vi "Unit Test.vi"() -> ()   [LabVIEW 2019, in "Allmotion.lvlib"]
uses:
  Allmotion.lvlib
  User Event/Controls/UE Abort Action.ctl
panel:
  in  "Open":bool
  out "Event":string
  in  "Current Position":i32[](array[numeric])
  in  "EMC Stop":bool
  in  "Joystick":bool
  in  "Reset":bool
  in  "Position":bool
  in  "Move":bool
  in  "Home":bool
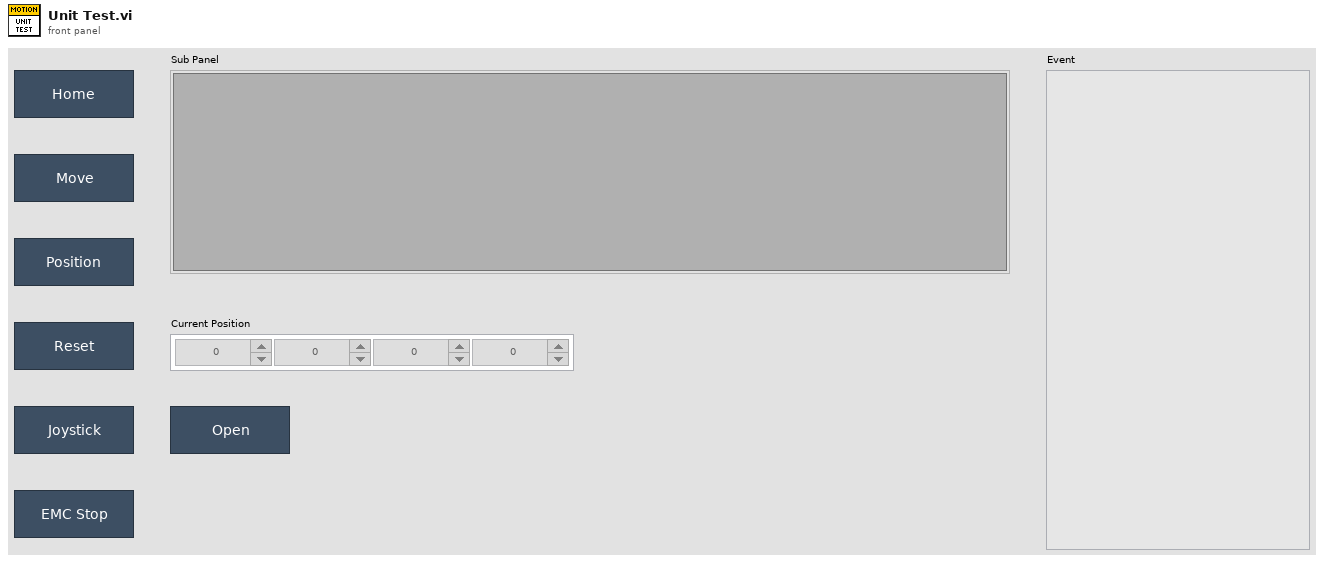
[diagram p1: front panel]
types:
  T1 = cluster{"Position":i32[], "Event":string, "Control Ref":refnum<vi>}
  T2 = typedef "UE Abort Action.ctl" = enum16{"Create", "Get", "Destroy"}
  T3 = typedef "Allmotion.lvlib/SEQ Data.ctl" = cluster{"Position":i32[], "Arrived?":bool, "VISA name":refnum<visa-resource-name>, "Initialize Done?":bool, "State":string, "VI Refnum":refnum<vi>, "Dichroic Position":string[]}
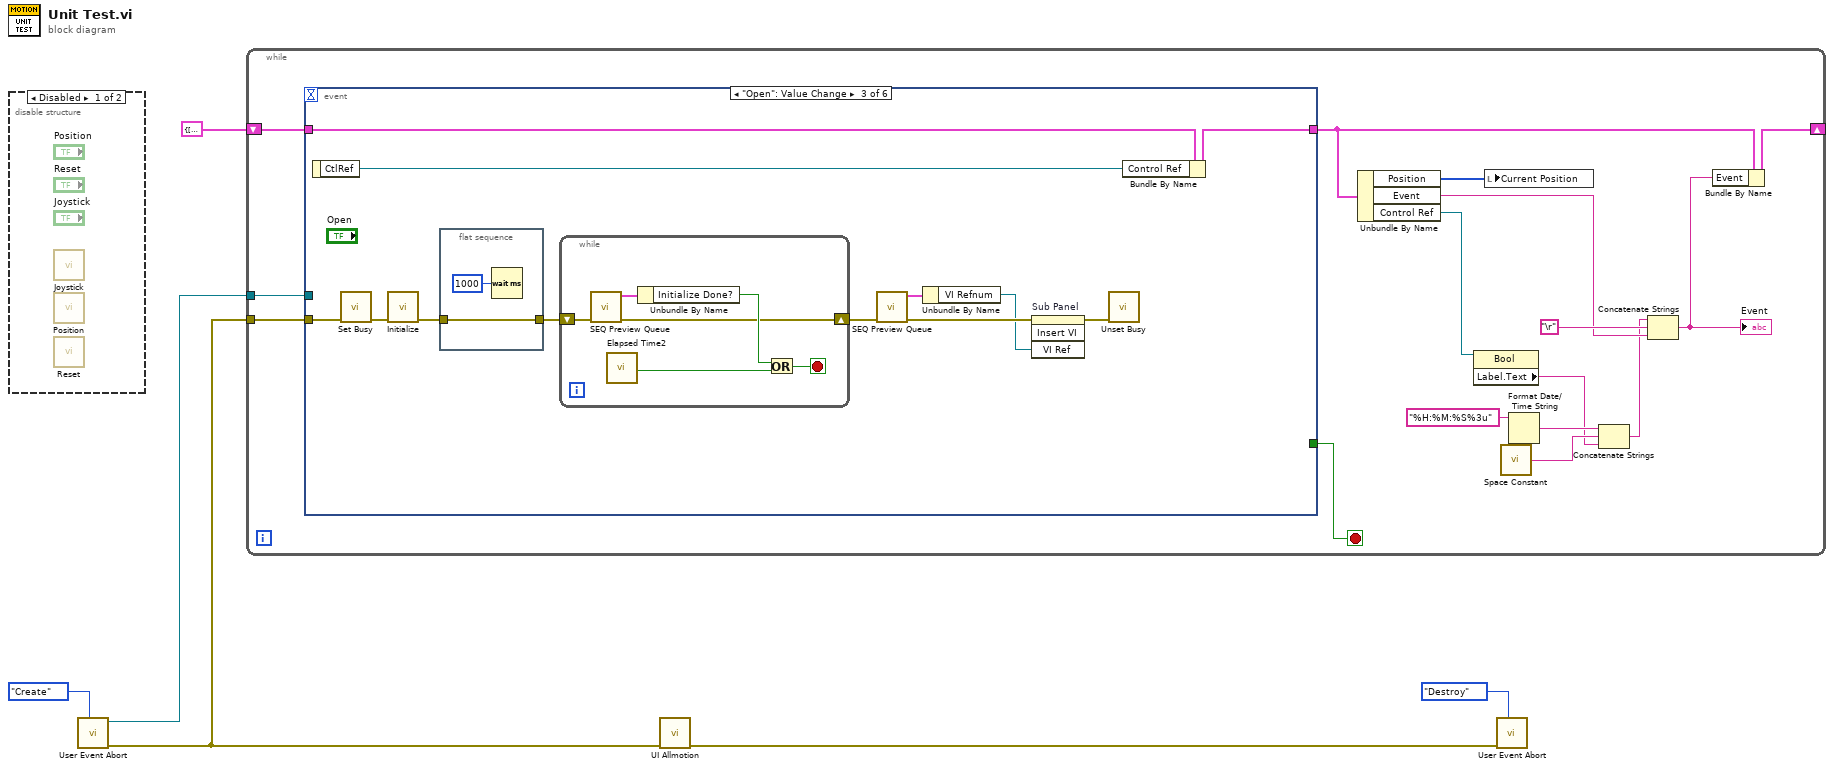
[diagram p0: block diagram]
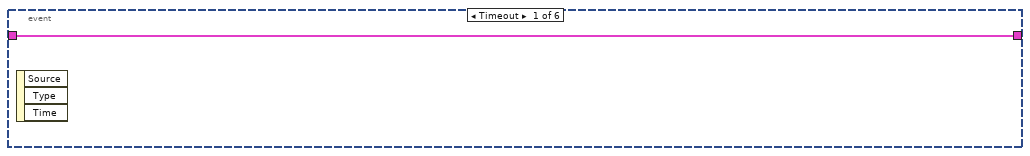
[diagram p3: hidden frame]
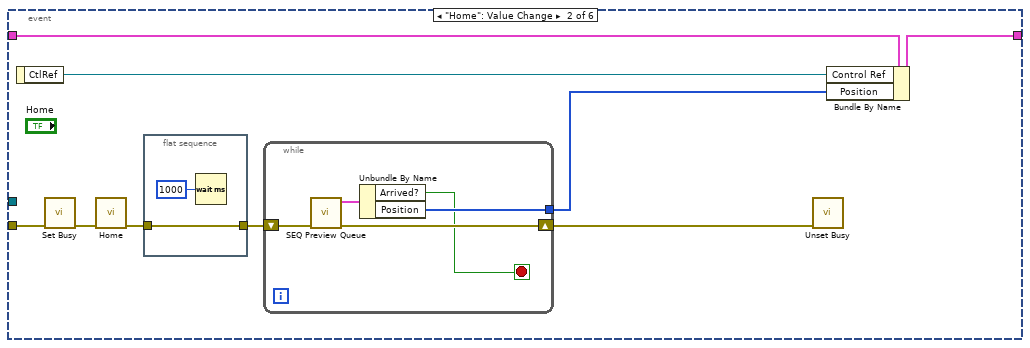
[diagram p4: hidden frame]
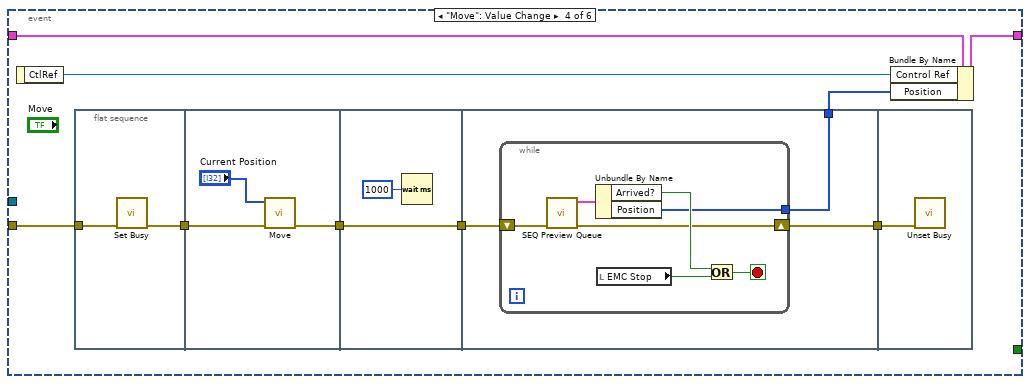
[diagram p5: hidden frame]
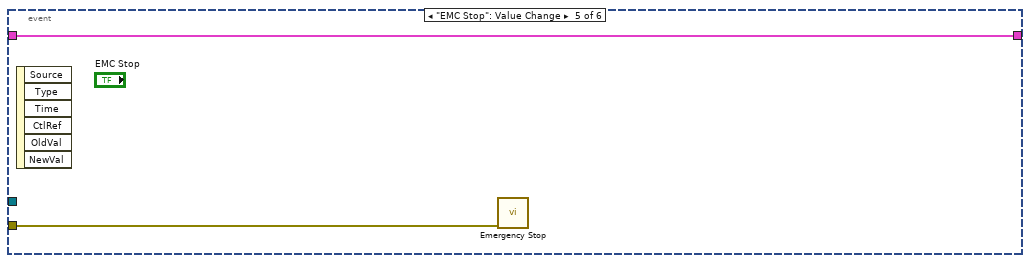
[diagram p6: hidden frame]
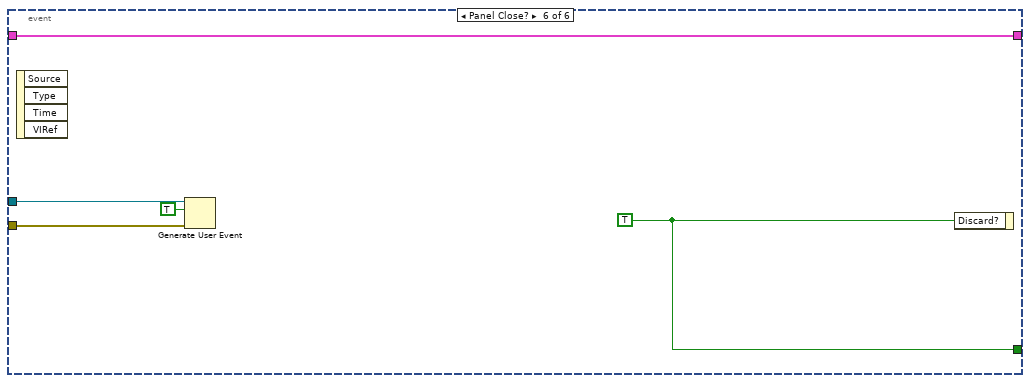
[diagram p7: hidden frame]
diagram:
  n1 = disable-structure shown="Disabled" {
    frame Disabled {
      n2 = call "Joystick.vi"() -> ()  [unwired: 11 in, 1 out]
      n3 = call "Position.vi"() -> ()  [unwired: 11 in, 1 out]
      n4 = call "Reset.vi"() -> ()  [unwired: 11 in, 1 out]
    }
    frame Enabled {
    }
  }
  n5 = call "User Event Abort.vi"("Action"=UE_Abort_Action."Create") -> ("Error Out"=w4:errorcluster, "User Event Out"=w5:refnum<user-event>)  [unwired: 9 in]
  n6 = while {
    tunnel: w5 -> [w21]
    tunnel: w4 -> [w20]
    shift-right: [w15] -> _
    shift-left: T1 {"Position"=[], "Event"="", "Control Ref"=refnum} -> [w19]
    stop <- w22 stop-if-true
    n7 = event shown="[2] \"Open\": Value Change" {
      selector: _ -> [_ _ _ _ _ _]
      dyn-events: _ -> [_ _ _ _ _ _]
      timeout: _ -> [_ _ _ _ _ _]
      tunnel: [_ _ _ _ _ w93] -> w22
      tunnel: w21 -> [_ _ _ _ _ w92]
      tunnel: w20 -> [_ w32 w51 w68 w87 w90]
      tunnel: w19 -> [w23 w30 w50 w64 w88 w89]
      tunnel: [w23 w29 w49 w63 w88 w89] -> w18
      event Timeout {
        n8 = event-data() -> ()  [unwired: 1 in, 3 out]
      }
      event "Home": Value Change {
        n9 = event-data() -> ("CtlRef"=w28:refnum<vi>)  [unwired: 1 in]
        n10 = call <vilib>:"Set Busy.vi"("error in (no error)"=w32) -> ("error out"=w31:errorcluster)  [unwired: 9 in, 1 out]
        n11 = call "Home.vi"("Error In"=w31) -> ("Error Out"=w26:errorcluster)  [unwired: 10 in]
        n12 = flat-sequence {
          tunnel: w26 -> [w33]
          tunnel: [w33] -> w25
          frame #0 {
            n13 = Wait (ms)(milliseconds to wait=u32 1000) -> ()  [unwired: 1 out]
          }
        }
        n14 = while {
          tunnel: [w37] -> w27
          shift-right: [w36] -> w24
          shift-left: w25 -> [w39]
          stop <- w35 stop-if-true
          n15 = call "SEQ Preview Queue.vi"("error in"=w39) -> ("error out"=w36:errorcluster, "SEQ Data"=w38:T3)  [unwired: 9 in]
          n16 = Unbundle By Name(w38) -> ("Arrived?"=w35:bool, "Position"=w37:i32[])
        }
        n17 = call <vilib>:"Unset Busy.vi"("error in (no error)"=w24) -> ()  [unwired: 10 in, 1 out]
        n18 = Bundle By Name(cluster=w30, "Control Ref"=w28, "Position"=w27) -> (w29:T1)
      }
      event "Open": Value Change {
        n19 = event-data() -> ("CtlRef"=w48:refnum<vi>)  [unwired: 1 in]
        n20 = call <vilib>:"Set Busy.vi"("error in (no error)"=w51) -> ("error out"=w42:errorcluster)  [unwired: 9 in, 1 out]
        n21 = call "Initialize.vi"("Error In"=w42) -> ("Error Out"=w41:errorcluster)  [unwired: 10 in]
        n22 = flat-sequence {
          tunnel: w41 -> [w52]
          tunnel: [w52] -> w40
          frame #0 {
            n23 = Wait (ms)(milliseconds to wait=u32 1000) -> ()  [unwired: 1 out]
          }
        }
        n24 = while {
          shift-right: [w55] -> w47
          shift-left: w40 -> [w59]
          stop <- w57 stop-if-true
          n25 = call "SEQ Preview Queue.vi"("error in"=w59) -> ("error out"=w55:errorcluster, "SEQ Data"=w58:T3)  [unwired: 9 in]
          n26 = call "Elapsed Time2"() -> ("Time has Elapsed"=w54:bool)  [unwired: 12 in, 7 out]
          n27 = Unbundle By Name(w58) -> ("Initialize Done?"=w56:bool)
          n28 = Or(x=w56, y=w54) -> (x .or. y?=w57:bool)
        }
        n29 = call "SEQ Preview Queue.vi"("error in"=w47) -> ("error out"=w45:errorcluster, "SEQ Data"=w46:T3)  [unwired: 9 in]
        n30 = Unbundle By Name(w46) -> ("VI Refnum"=w43:refnum<vi>)
        n31 = invoke on="Sub Panel" class="SubPnl" method="Insert VI"(error in=w45, "VI Ref"=w43) -> (error out=w44:errorcluster)  [unwired: 2 in, 3 out]
        n32 = call <vilib>:"Unset Busy.vi"("error in (no error)"=w44) -> ()  [unwired: 10 in, 1 out]
        n33 = Bundle By Name(cluster=w50, "Control Ref"=w48) -> (w49:T1)
      }
      event "Move": Value Change {
        n34 = event-data() -> ("CtlRef"=w62:refnum<vi>)  [unwired: 1 in]
        n35 = flat-sequence {
          tunnel: w68 -> [w70]
          tunnel: [w69] -> w67
          tunnel: w67 -> [w73]
          tunnel: [w72] -> w66
          tunnel: w66 -> [w75]
          tunnel: [w75] -> w65
          tunnel: w65 -> [w78]
          tunnel: [w76] -> w61
          tunnel: [w77] -> w60
          tunnel: w60 -> [w86]
          frame #0 {
            n36 = call <vilib>:"Set Busy.vi"("error in (no error)"=w70) -> ("error out"=w69:errorcluster)  [unwired: 9 in, 1 out]
          }
          frame #1 {
            n37 = call "Move.vi"("Error In"=w73, "Target Position"="Current Position") -> ("Error Out"=w72:errorcluster)  [unwired: 9 in]
          }
          frame #2 {
            n38 = Wait (ms)(milliseconds to wait=u32 1000) -> ()  [unwired: 1 out]
          }
          frame #3 {
            n39 = while {
              tunnel: [w80] -> w76
              shift-right: [w79] -> w77
              shift-left: w78 -> [w85]
              stop <- w83 stop-if-true
              n40 = call "SEQ Preview Queue.vi"("error in"=w85) -> ("error out"=w79:errorcluster, "SEQ Data"=w84:T3)  [unwired: 9 in]
              n41 = Unbundle By Name(w84) -> ("Arrived?"=w81:bool, "Position"=w80:i32[])
              n42 = local read "EMC Stop"() -> (w82:bool)
              n43 = Or(x=w81, y=w82) -> (x .or. y?=w83:bool)
            }
          }
          frame #4 {
            n44 = call <vilib>:"Unset Busy.vi"("error in (no error)"=w86) -> ()  [unwired: 10 in, 1 out]
          }
        }
        n45 = Bundle By Name(cluster=w64, "Control Ref"=w62, "Position"=w61) -> (w63:T1)
      }
      event "EMC Stop": Value Change {
        n46 = event-data() -> ()  [unwired: 1 in, 6 out]
        n47 = call "Emergency Stop.vi"("Error In"=w87) -> ()  [unwired: 10 in, 1 out]
      }
      event Panel Close? {
        w93 = TRUE ("Discard?")
        n48 = event-data() -> ()  [unwired: 1 in, 4 out]
        n49 = Generate User Event(user event=w92, event data cluster=TRUE ("event data"), error in=w90) -> ()  [unwired: 1 in, 2 out]
        n50 = event-data("Discard?"=w93) -> ()  [unwired: 1 in, 1 out]
      }
    }
    n51 = Unbundle By Name(w18) -> ("Position"=w17:i32[], "Event"=w13:string, "Control Ref"=w16:refnum<vi>)
    n52 = property class="Bool"(reference=w16) -> ("Label.Text"=w8:string)  [unwired: 1 in, 2 out]
    n53 = local write "Current Position"(w17) -> ()
    n54 = call <vilib>:"Space Constant.vi"() -> ("String"=w9:string)
    n55 = Format Date/Time String(time format string (%c)="%H:%M:%S%3u") -> (date/time string=w10:string)  [unwired: 2 in]
    n56 = Concatenate Strings(w10, w9, w8) -> (w7:string)
    n57 = Concatenate Strings(w7, "\r", w13) -> (w12:string)
    "Event" <- w12
    n58 = Bundle By Name(cluster=w18, "Event"=w12) -> (w15:T1)
  }
  n59 = call "UI Allmotion.vi"("error in"=w4) -> ("error out"=w3:errorcluster)  [unwired: 10 in]
  n60 = call "User Event Abort.vi"("Action"=UE_Abort_Action."Destroy", "Error In"=w3) -> ()  [unwired: 8 in, 2 out]
